vi "Add TimeStamps.vi"(9 "TIme2":timestamp=timestamp(-19636 s since 1904-01-01) format="%<%H:%M:%S>T", 11 "Time1":timestamp=timestamp(-16030 s since 1904-01-01) format="%<%H:%M:%S>T") -> (1 "Resultant Time":timestamp format="%<%H:%M:%S>T")   [LabVIEW 2017]
doc: "AMEE"
panel:
  out "resulting string":string
  out "FInal Min":i32 format="%02d"
  out "Final Hr":i32 format="%02d"
  out "Final Seconds":i32
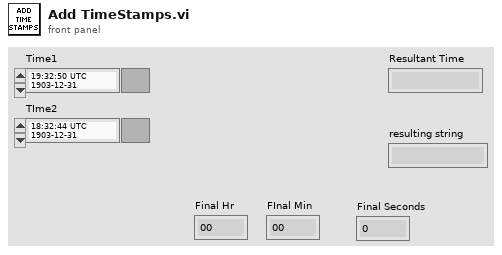
[diagram p1: front panel]
types:
  T1 = typedef "LVDateTimeRec.ctl" = cluster{"fractional second":dbl, "second":i32, "minute":i32, "hour":i32, "day of month":i32, "month":i32, "year":i32, "day of week":i32, "day of year":i32, "DST":i32}
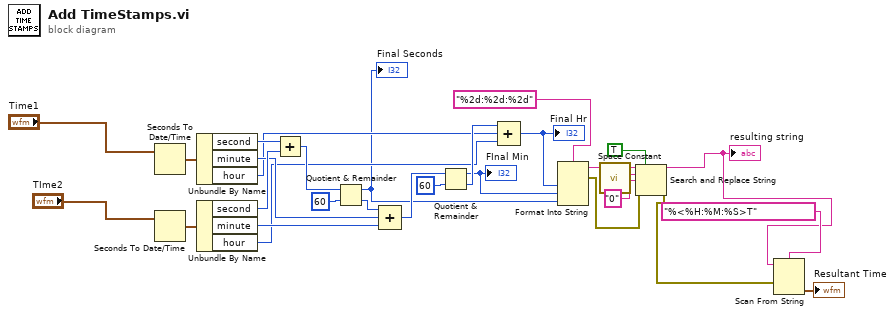
[diagram p0: block diagram]
diagram:
  n1 = Seconds To Date/Time(time stamp (now)="Time1") -> (date time rec=w27:T1)  [unwired: 1 in]
  n2 = Seconds To Date/Time(time stamp (now)="TIme2") -> (date time rec=w28:T1)  [unwired: 1 in]
  n3 = Unbundle By Name(w27) -> ("second"=w25:i32, "minute"=w21:i32, "hour"=w15:i32)
  n4 = Unbundle By Name(w28) -> ("second"=w24:i32, "minute"=w20:i32, "hour"=w14:i32)
  n5 = Add(x=w25, y=w24) -> (x+y=w23:i32)
  n6 = Quotient & Remainder(x=w23, y=60) -> (x-y*floor(x/y)=w10:i32, floor(x/y)=w19:i32)
  "Final Seconds" <- w10
  n7 = Compound Arithmetic op=ADD(w19, w21, w20) -> (w18:i32)
  n8 = Quotient & Remainder(x=w18, y=60) -> (x-y*floor(x/y)=w11:i32, floor(x/y)=w16:i32)
  "FInal Min" <- w11
  n9 = Compound Arithmetic op=ADD(w16, w15, w14) -> (w12:i32)
  "Final Hr" <- w12
  n10 = Format Into String(format string="%2d:%2d:%2d", w12, w11, w10) -> (resulting string=w9:string, error out=w2:errorcluster)  [unwired: 2 in]
  n11 = call <vilib>:"Space Constant.vi"() -> ("String"=w8:string)
  n12 = Search and Replace String(replace all?=TRUE ("replace all? (F)"), input string=w9, search string=w8, replace string="0" ("replace string (\"\")"), error in=w2) -> (result string=w4:string, error out=w1:errorcluster)  [unwired: 3 in, 2 out]
  "resulting string" <- w4
  n13 = Scan From String(format string="%<%H:%M:%S>T", input string=w4, error in=w1) -> (output 1=→"Resultant Time":timestamp)  [unwired: 2 in, 3 out]
